vi "Scroll Textfield to Bottom.vi"(6 "Console String":refnum<vi>, 8 "error in (no error)":errorcluster, 10 "Bytes at Serial Port":u32, 11 "VISA refnum in":refnum<visa-resource-name>) -> (0 "error out":errorcluster, 3 "VISA refnum out":refnum<visa-resource-name>)   [LabVIEW 2024]
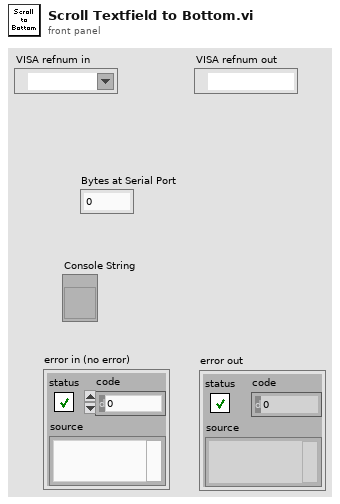
[diagram p1: front panel]
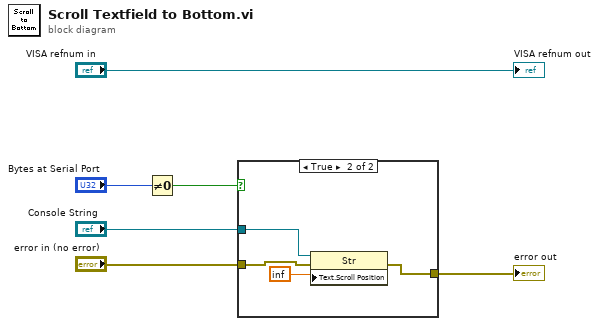
[diagram p0: block diagram]
diagram:
  n1 = Not Equal To 0?(x="Bytes at Serial Port") -> (x != 0?=w4:bool)
  n2 = case shown="True" w4 {
    tunnel: [w7 w10] -> w3
    tunnel: "error in (no error)" -> [w7 w9]
    tunnel: "Console String" -> [_ w8]
    frame False {
    }
    frame True {
      n3 = property class="Str"(reference=w8, error in=w9, "Text.Scroll Position"=inf) -> (error out=w10:errorcluster)  [unwired: 1 out]
    }
  }
  "error out" <- w3
  "VISA refnum out" <- "VISA refnum in"
